vi "read_tcx_file.vi"(8 "error in":errorcluster, 11 "File Path":path) -> (0 "error out":errorcluster, 2 "Time":timestamp[](array[timestamp]), 3 "Bmp":i32[](array[numeric]))   [LabVIEW 2025]
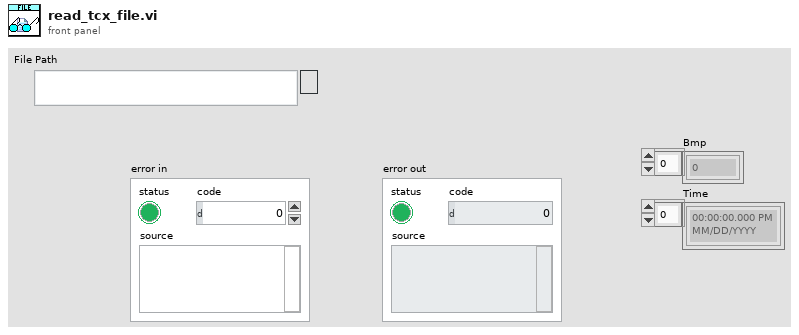
[diagram p1: front panel]
types:
  T1 = enum16{"open", "replace", "create", "open or create", "replace or create", "replace or create with confirmation"}
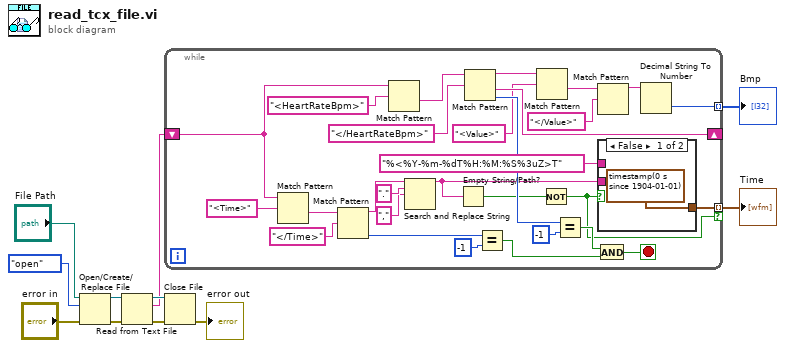
[diagram p0: block diagram]
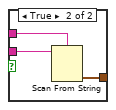
[diagram p2: hidden frame]
diagram:
  n1 = Open/Create/Replace File(file path (use dialog)="File Path", error in="error in", operation (0:open)=T1."open") -> (refnum out=w5:refnum<file>, error out=w9:errorcluster)  [unwired: 3 in, 1 out]
  n2 = Read from Text File(file (use dialog)=w5, error in=w9) -> (refnum out=w4:refnum<file>, text=w3:string, error out=w8:errorcluster)  [unwired: 2 in, 1 out]
  n3 = while {
    shift-right: [w38] -> _
    shift-left: w3 -> [w28]
    tunnel: [w29] -> w2 mode=indexing
    tunnel: [w13] -> w1 mode=indexing if=w12
    stop <- w19 stop-if-true
    n4 = Match Pattern(string=w28, regular expression="<Time>") -> (after substring=w25:string)  [unwired: 1 in, 3 out]
    n5 = Match Pattern(string=w25, regular expression="</Time>") -> (before substring=w22:string, offset past match=w24:i32)  [unwired: 1 in, 2 out]
    n6 = Match Pattern(string=w28, regular expression="<HeartRateBpm>") -> (after substring=w30:string)  [unwired: 1 in, 3 out]
    n7 = Search and Replace String(input string=w22, search string=".", replace string="," ("replace string (\"\")")) -> (result string=w14:string)  [unwired: 5 in, 3 out]
    n8 = Empty String/Path?(string/path=w14) -> (empty?=w16:bool)
    n9 = Match Pattern(string=w30, regular expression="</HeartRateBpm>") -> (before substring=w31:string, after substring=w38:string, offset past match=w37:i32)  [unwired: 1 in, 1 out]
    n10 = Equal?(x=w24, y=-1) -> (x = y?=w17:bool)
    n11 = Match Pattern(string=w31, regular expression="<Value>") -> (after substring=w34:string)  [unwired: 1 in, 3 out]
    n12 = Not(x=w16) -> (.not. x?=w12:bool)
    n13 = Equal?(x=w37, y=-1) -> (x = y?=w18:bool)
    n14 = And(x=w18, y=w17) -> (x .and. y?=w19:bool)
    n15 = Match Pattern(string=w34, regular expression="</Value>") -> (before substring=w32:string)  [unwired: 1 in, 3 out]
    n16 = case shown="False" w12 {
      tunnel: "%<%Y-%m-%dT%H:%M:%S%3uZ>T" ("format string") -> [_ w44]
      tunnel: w14 -> [_ w43]
      tunnel: [timestamp(0 s since 1904-01-01) w42] -> w13
      frame False {
      }
      frame True {
        n17 = Scan From String(format string=w44, input string=w43) -> (output 1=w42:timestamp)  [unwired: 3 in, 3 out]
      }
    }
    n18 = Decimal String To Number(string=w32) -> (number=w29:i32)  [unwired: 2 in, 1 out]
  }
  "Bmp" <- w2
  "Time" <- w1
  n19 = Close File(refnum=w4, error in=w8) -> (error out=→"error out":errorcluster)  [unwired: 1 out]
